vi "Destroy.vi"(8 "error in (no error)":errorcluster, 11 "LV RT in":refnum<class "LV RT.lvclass">) -> (0 "error out":errorcluster, 3 "LV RT out":refnum<class "LV RT.lvclass">)   [LabVIEW 2016, in "LV RT.lvclass"]
uses:
  LV RT.lvclass
  D:/Navin Workspace/MDI/source code/Document/LV Doc/LV Doc.lvclass
  LV Doc.lvclass/LV Doc.ctl
  LV RT.lvclass/LV RT.ctl
  property/Read VI Reference.vi
  property/Read Instantiated by ref_.vi
  LV Doc.lvclass
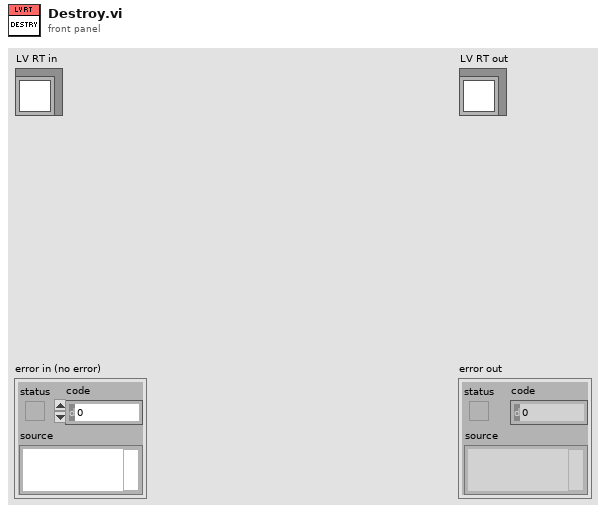
[diagram p1: front panel]
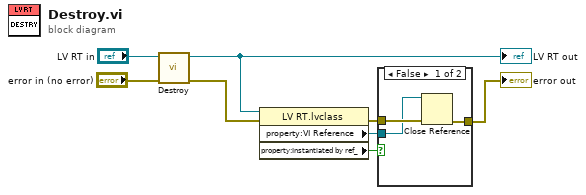
[diagram p0: block diagram]
diagram:
  n1 = call-parent "Destroy.vi"("error in (no error)"="error in (no error)", "Document in"="LV RT in") -> ("error out"=w5:errorcluster, "Document out"=w6:refnum<class "LV RT.lvclass">)  [unwired: 8 in]
  "LV RT out" <- w6
  n2 = property class="LV RT.lvclass"(reference=w6, error in=w5) -> (error out=w4:errorcluster, "property:VI Reference"=w3:refnum<vi>, "property:Instantiated by ref_"=w1:bool)  [unwired: 1 out]
  n3 = case shown="False" w1 {
    tunnel: w4 -> [w11 w12]
    tunnel: w3 -> [w10 _]
    tunnel: [w9 w12] -> w2
    frame False {
      n4 = Close Reference(reference=w10, error in (no error)=w11) -> (error out=w9:errorcluster)
    }
    frame True {
    }
  }
  "error out" <- w2
